vi "Calc Long Word Padded Width (excel).vi"(1 "bit depth":i32, 2 "width":i32) -> (0 "padded width":i32)   [LabVIEW 2020, in "NI_ReportGenerationToolkit.lvlib"]
doc: "This VI calculates the byte width of one row of a bitmap in Windows BMP file format. BMP bitmaps should be padded so that each row begins on a 32 bit boundary."
uses:
  <vilib>/addons/_office/NI_ReportGenerationToolkit.lvlib
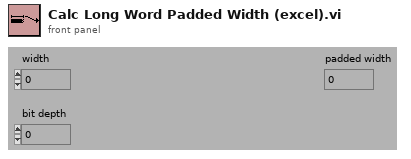
[diagram p1: front panel]
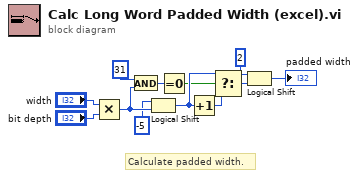
[diagram p0: block diagram]
diagram:
  # "Calculate padded width."
  n1 = Multiply(x="width", y="bit depth") -> (x*y=w5:i32)
  n2 = And(x=31, y=w5) -> (x .and. y?=w7:i32)
  n3 = Logical Shift(y=-5, x=w5) -> (x << y=w9:i32)
  n4 = Equal To 0?(x=w7) -> (x = 0?=w8:bool)
  n5 = Increment(x=w9) -> (x+1=w10:i32)
  n6 = Select(t=w9, s=w8, f=w10) -> (s? t:f=w12:i32)
  n7 = Logical Shift(y=2, x=w12) -> (x << y=→"padded width":i32)
